vi "ke2000 Revision Query.vi"(0 "VISA resource name":refnum<visa-resource-name>, 5 "error in (no error)":errorcluster) -> (14 "VISA resource name out":refnum<visa-resource-name>, 17 "Instr Driver Revision":string, 18 "Instr Firmware Revision":string, 19 "error out":errorcluster)   [LabVIEW 2010]
doc: "This VI queries the current instrument firmware revision and instrument driver revision.\n\nThis Instrument Driver's Revision number is 2.0 and is compatible with Instrument Firmware Revision A13/A02.\n\nke2000\nCreated By: National Instruments (Adam Kemp)\nRelease Date: 11/03\nOriginally Developed in LabVIEW Version: 7.0\n\nModification History:\n\nREV 1.0, 01/1995\nOriginal Release.\n\nREV 2.0, 11/2003, LV 7.0\nCreated by: Adam Kemp, NI\nRewrote Driver to include major API updates and to make consistant with current instrument driver guidelines. Version 2.0 and above are not backward compatible with version 1.x\n\nREV 2.1, 10/2004, LV 7.0\nUpdated by: Matthew McClintock, NI\n- Configure an immeadiate trigger in the Default Instrument Setup VI\n- Reordered the sequence of commands in Wait for SRQ to avoid race conditions"
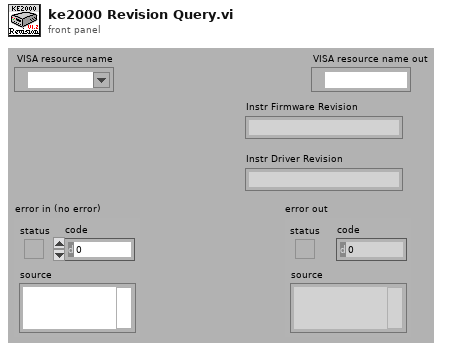
[diagram p1: front panel]
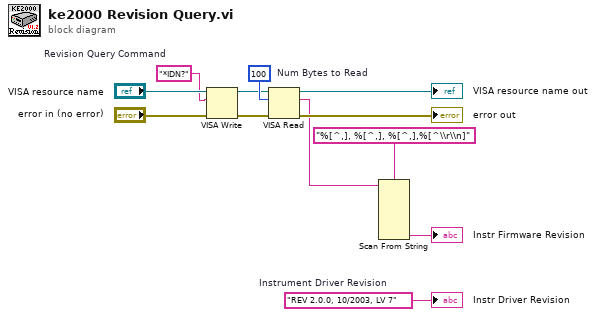
[diagram p0: block diagram]
diagram:
  w3 = "*IDN?"  # Revision Query Command
  w6 = u32 100  # Num Bytes to Read
  w12 = "REV 2.0.0, 10/2003, LV 7"  # Instrument Driver Revision
  n1 = VISA Write(VISA resource name="VISA resource name", write buffer=w3, error in (no error)="error in (no error)") -> (VISA resource name out=w5:refnum<visa-resource-name>, error out=w4:errorcluster)  [unwired: 1 out]
  n2 = VISA Read(VISA resource name=w5, byte count=w6, error in (no error)=w4) -> (VISA resource name out=→"VISA resource name out":refnum<visa-resource-name>, read buffer=w2:string, error out=→"error out":errorcluster)  [unwired: 1 out]
  n3 = Scan From String(format string="%[^,], %[^,], %[^,],%[^\\r\\n]", input string=w2) -> (output 4=→"Instr Firmware Revision":string)  [unwired: 9 in, 3 out]
  "Instr Driver Revision" <- w12
